vi "SP Convert SPs to TPs.vi"(10 "SP Array":T1) -> (2 "T-Parameters":T2)   [LabVIEW 2011]
uses:
  TypeDefs/SP TP Data.ctl
  TypeDefs/SP Data.ctl
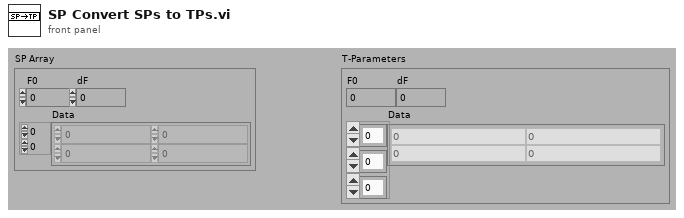
[diagram p1: front panel]
types:
  T1 = typedef "SP Data.ctl" = cluster{"F0":dbl, "dF":dbl, "Data":cdb[][]}
  T2 = typedef "SP TP Data.ctl" = cluster{"F0":dbl, "dF":dbl, "Data":cdb[][][]}
  T3 = typedef "SP Complex Matrix.ctl" = cdb[][]
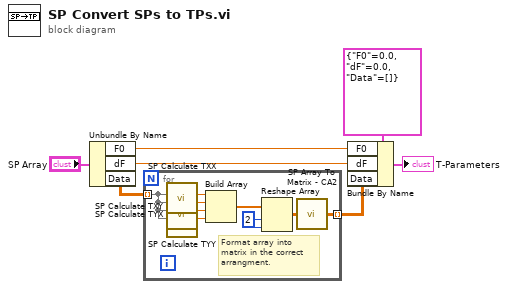
[diagram p0: block diagram]
diagram:
  n1 = Unbundle By Name("SP Array") -> ("F0"=w1:dbl, "dF"=w2:dbl, "Data"=w6:cdb[][])
  n2 = for {
    tunnel: w6 -> [w8] mode=indexing
    tunnel: [w15] -> w4 mode=indexing
    w16 = 2 ("dimension size")
    # "Format array into\nmatrix in the correct\narrangment."
    n3 = call "SP Calculate TXX.vi"("SP Array (SXX, SXY, SYX, SYY)"=w8) -> ("TXX"=w12:cdb)  [unwired: 10 out]
    n4 = call "SP Calculate TXY.vi"("SP Array (SXX, SXY, SYX, SYY)"=w8) -> ("TXY"=w11:cdb)  [unwired: 10 out]
    n5 = call "SP Calculate TYX.vi"("SP Array (SXX, SXY, SYX, SYY)"=w8) -> ("TYX"=w10:cdb)  [unwired: 10 out]
    n6 = call "SP Calculate TYY.vi"("SP Array (SXX, SXY, SYX, SYY)"=w8) -> ("TYY"=w9:cdb)  [unwired: 10 out]
    n7 = Build Array(w12, w11, w10, w9) -> (w13:cdb[])
    n8 = Reshape Array(w13, w16, w16) -> (w14:cdb[][])
    n9 = call "SP Array To Matrix - CA2.vi"("Complex 2D Array"=w14) -> ("Complex Matrix"=w15:T3)
  }
  n10 = Bundle By Name(cluster=T2 {"F0"=0.0, "dF"=0.0, "Data"=[]} ("T-Parameters"), "F0"=w1, "dF"=w2, "Data"=w4) -> (→"T-Parameters":T2)
